vi "9233_Initialize.vi"(8 "error in (no error)":errorcluster, 9 "Slot Settings":T1, 11 "9233 in":refnum<class "9233.lvclass">) -> (0 "error out":errorcluster, 3 "9233 out":refnum<class "9233.lvclass">)   [LabVIEW 2019, in "Modules.lvlib" / "9233.lvclass"]
uses:
  9233.lvclass
  RSI Module/Slot Settings.ctl
  C:/Users/nitest/Desktop/Git 2019/niveristand-scan-engine-module-libraries/Source/RSI Module/RSI Module.lvclass
  RSI Module/Channels.ctl
  RSI Module/Channel Type.ctl
  RSI Module/Module Models.ctl
  Data rate.ctl
  9233.lvclass/9233.ctl
  RSI Module/RSI Module.lvclass
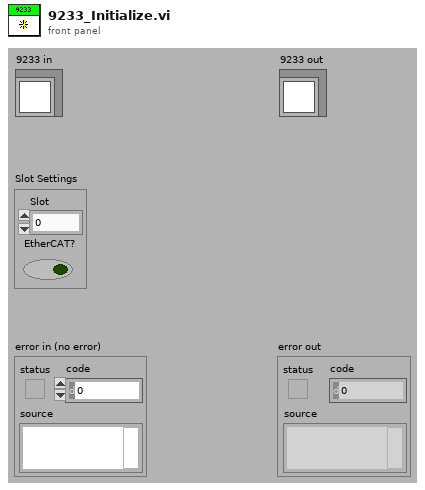
[diagram p1: front panel]
types:
  T1 = typedef "Modules.lvlib/RSI Module.lvclass/Slot Settings.ctl" = cluster{"Slot":u32, "EtherCAT?":bool}
  T2 = typedef "Modules.lvlib/RSI Module.lvclass/Module Models.ctl" = enum16{"Empty", "NI 9201", "NI 9203", "NI 9205", "NI 9206", "NI 9207", "NI 9208", "NI 9209", "NI 9210", "NI 9211", "NI 9212", "NI 9213", "NI 9214", "NI 9215", "NI 9216", "NI 9217", "NI 9219", "NI 9220", "NI 9221", "NI 9222", "NI 9223", "NI 9224", "NI 9225", "NI 9226", "NI 9227", "NI 9228", "NI 9229", "NI 9233", "NI 9234", "NI 9235", "NI 9236", "NI 9237", "NI 9239", "NI 9242", "NI 9244", "NI 9253", "NI 9263", "NI 9264", "NI 9265", "NI 9266", "NI 9269", "NI 9344", "NI 9350", "NI 9375", "NI 9401", "NI 9402", "NI 9403", "NI 9411", "NI 9421", "NI 9422", "NI 9423", "NI 9425", "NI 9426", "NI 9435", "NI 9436", "NI 9437", "NI 9472", "NI 9474", "NI 9475", "NI 9476", "NI 9477", "NI 9478", "NI 9481", "NI 9482", "NI 9485"}
  T3 = typedef "Modules.lvlib/RSI Module.lvclass/Channels.ctl" = cluster{"# Input Channels":i32, "# Output Channels":i32, "Channel Type":T4, "Units":string}
  T4 = typedef "Modules.lvlib/RSI Module.lvclass/Channel Type.ctl" = enum16{"Analog", "Digital"}
  T5 = typedef "Modules.lvlib/9233.lvclass/Data rate.ctl" = u32
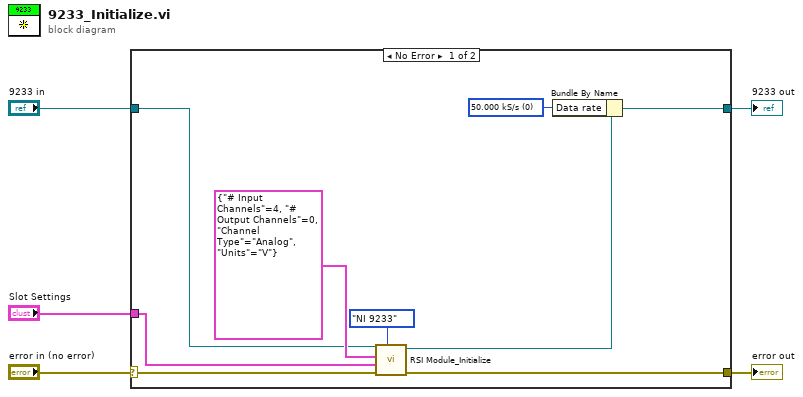
[diagram p0: block diagram]
diagram:
  n1 = case shown="No Error" "error in (no error)" {
    selector: "error in (no error)" -> [w11 w16]
    tunnel: [w10 w16] -> w4
    tunnel: [w8 w15] -> w2
    tunnel: "9233 in" -> [w13 w15]
    tunnel: "Slot Settings" -> [w12 _]
    frame No Error {
      w6 = T5 0 items=["50.000 kS/s", "25.000 kS/s", "16.667 kS/s", "12.500 kS/s", "10.000 kS/s", "8.333 kS/s", "7.143 kS/s", "6.250 kS/s", "5.556 kS/s", "5.000 kS/s", "4.545 kS/s", "4.167 kS/s", "3.846 kS/s", "3.571 kS/s", "3.333 kS/s", "3.125 kS/s", "2.941 kS/s", "2.778 kS/s", "2.632 kS/s", "2.500 kS/s", "2.381 kS/s", "2.273 kS/s", "2.174 kS/s", "2.083 kS/s", "2.000 kS/s", "1.923 kS/s", "1.852 kS/s", "1.786 kS/s", "1.724 kS/s", "1.667 kS/s", "1.613 kS/s"] ("Data rate")
      n2 = call "RSI Module_Initialize.vi"("Module Model"=Module_Models."NI 9233", "error in (no error)"=w11, "Slot Settings"=w12, "Channels"=T3 {"# Input Channels"=4, "# Output Channels"=0, "Channel Type"=enum."Analog", "Units"="V"}, "RSI Module in"=w13) -> ("error out"=w10:errorcluster, "RSI Module out"=w9:refnum<class "9233.lvclass">)  [unwired: 5 in]
      n3 = Bundle By Name(cluster=w9, "Data rate"=w6) -> (w8:refnum<class "9233.lvclass">)
    }
    frame Error {
    }
  }
  "error out" <- w4
  "9233 out" <- w2
